vi "Subtractor4.vi"() -> (8 "Subtractor4":refnum<class "Subtractor4.lvclass">)   [LabVIEW 2017, in "Subtractor4.lvclass"]
uses:
  Subtractor4.lvclass
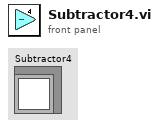
[diagram p1: front panel]
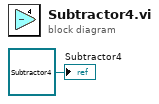
[diagram p0: block diagram]
diagram:
  "Subtractor4" <- refnum<class "Subtractor4.lvclass"> refnum ("Subtractor4.lvclass")
